vi "GV frame gate.vi"() -> ()   [LabVIEW 2017]
panel:
  out "Frame gate":bool
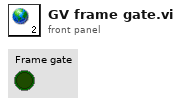
[diagram p1: front panel]
diagram:
